vi "Calibracion Elevador Global.vi"() -> ()   [LabVIEW 2014]
panel:
  in  "calibrar":bool
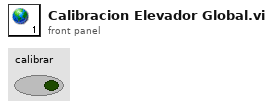
[diagram p1: front panel]
diagram:
